vi "Save-Recall Instrument Settings.vi"(8 "error in (no error)":errorcluster, 9 "State Identification":string, 10 "Operation (3:Save State)":u16(ring)=3 items=["Delete All", "Delete State", "Recall State", "Save State"], 11 "VISA resource name":refnum<visa-resource-name>) -> (0 "error out":errorcluster, 3 "VISA resource name out":refnum<visa-resource-name>)   [LabVIEW 2020, in "3458A Basic Driver.lvlib"]
doc: "Saves and Recalls different states of the instrument. This VI can also delete a state or all states from memory. Note that to recall a state, you must choose the \"load state\" function and type in the name of the state in the \"state identification\" control indicating which saved state you want to load."
uses:
  3458A Basic Driver.lvlib
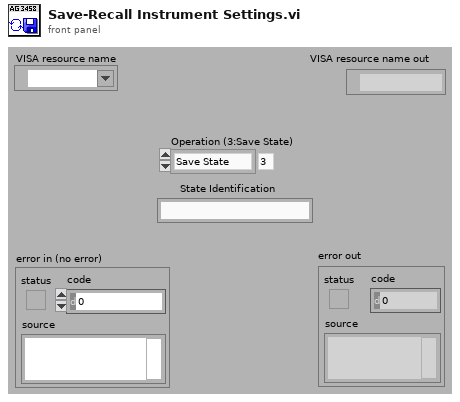
[diagram p1: front panel]
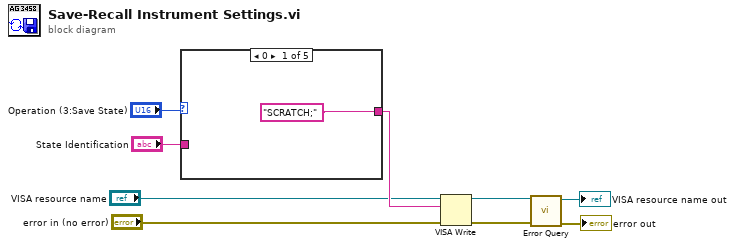
[diagram p0: block diagram]
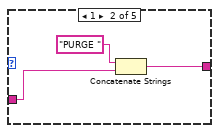
[diagram p2: hidden frame]
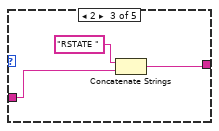
[diagram p3: hidden frame]
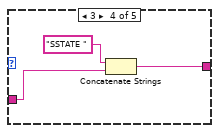
[diagram p4: hidden frame]
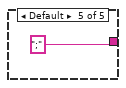
[diagram p5: hidden frame]
diagram:
  n1 = case shown="0" "Operation (3:Save State)" {
    tunnel: "State Identification" -> [_ w12 w15 w18 _]
    tunnel: ["SCRATCH;" w11 w14 w17 ";"] -> w9
    frame 0 {
    }
    frame 1 {
      n2 = Concatenate Strings("PURGE ", w12) -> (w11:string)
    }
    frame 2 {
      n3 = Concatenate Strings("RSTATE ", w15) -> (w14:string)
    }
    frame 3 {
      n4 = Concatenate Strings("SSTATE ", w18) -> (w17:string)
    }
    frame Default {
    }
  }
  n5 = VISA Write(VISA resource name="VISA resource name", write buffer=w9, error in (no error)="error in (no error)") -> (VISA resource name out=w8:refnum<visa-resource-name>, error out=w7:errorcluster)  [unwired: 1 out]
  n6 = call "Error Query.vi"("error in (no error)"=w7, "VISA resource name"=w8) -> ("error out"=→"error out":errorcluster, "VISA resource name out"=→"VISA resource name out":refnum<visa-resource-name>)  [unwired: 6 in, 2 out]
